vi "Analog_Output_16Channels_W20I5.vi"(1 "Values":fxp<+/-,20,5>[](array[numeric])=[0.0, 0.0, 0.0, 0.0, 0.0, 0.0, 0.0, 0.0, 0.0, 0.0, 0.0, 0.0, 0.0, 0.0, 0.0, 0.0], 2 "IO":T1={"AO 0"="Mod4/AO0", "AO 1"="Mod4/AO0", "AO 2"="Mod4/AO0", "AO 3"="Mod4/AO0", "AO 4"="Mod4/AO0", "AO 5"="Mod4/AO0", "AO 6"="Mod4/AO0", "AO 7"="Mod4/AO0", "AO 8"="Mod4/AO0", "AO 9"="Mod4/AO0", "AO 10"="Mod4/AO0", "AO 11"="Mod4/AO0", "AO 12"="Mod4/AO0", "AO 13"="Mod4/AO0", "AO 14"="Mod4/AO0", "AO 15"="Mod4/AO0"}) -> ()   [LabVIEW 2015]
uses:
  <vilib>/rvi/eio/common/nirviEmuTemplateMethod_errors.vi
  <vilib>/eio/EIONode/EIONode.xnode
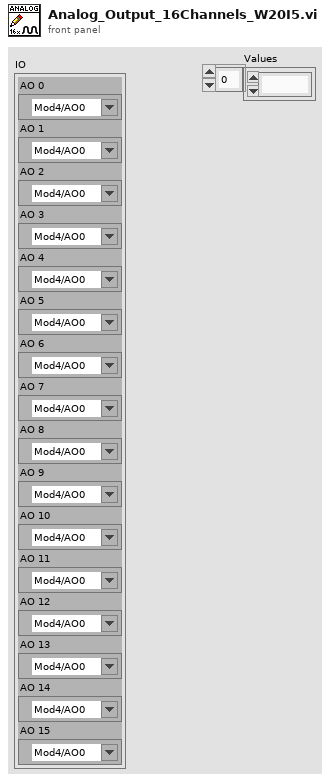
[diagram p1: front panel]
types:
  T1 = cluster{"AO 0":refnum<k21>, "AO 1":refnum<k21>, "AO 2":refnum<k21>, "AO 3":refnum<k21>, "AO 4":refnum<k21>, "AO 5":refnum<k21>, "AO 6":refnum<k21>, "AO 7":refnum<k21>, "AO 8":refnum<k21>, "AO 9":refnum<k21>, "AO 10":refnum<k21>, "AO 11":refnum<k21>, "AO 12":refnum<k21>, "AO 13":refnum<k21>, "AO 14":refnum<k21>, "AO 15":refnum<k21>}
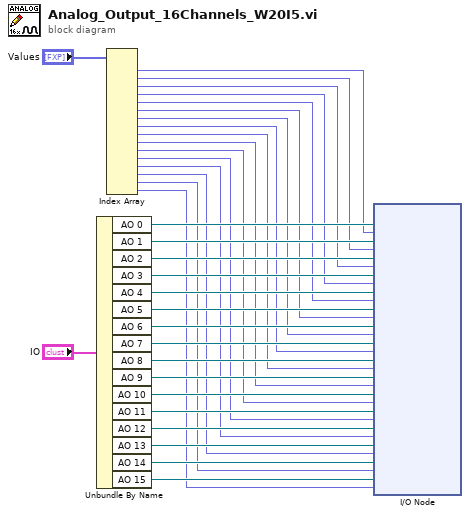
[diagram p0: block diagram]
diagram:
  n1 = Unbundle By Name("IO") -> ("AO 0"=w33:refnum<k21>, "AO 1"=w32:refnum<k21>, "AO 2"=w31:refnum<k21>, "AO 3"=w30:refnum<k21>, "AO 4"=w29:refnum<k21>, "AO 5"=w28:refnum<k21>, "AO 6"=w27:refnum<k21>, "AO 7"=w26:refnum<k21>, "AO 8"=w25:refnum<k21>, "AO 9"=w24:refnum<k21>, "AO 10"=w23:refnum<k21>, "AO 11"=w22:refnum<k21>, "AO 12"=w21:refnum<k21>, "AO 13"=w20:refnum<k21>, "AO 14"=w19:refnum<k21>, "AO 15"=w18:refnum<k21>)
  n2 = Index Array(array="Values") -> (element #1=w16:fxp<+/-,20,5>, element #2=w15:fxp<+/-,20,5>, element #3=w14:fxp<+/-,20,5>, element #4=w13:fxp<+/-,20,5>, element #5=w12:fxp<+/-,20,5>, element #6=w11:fxp<+/-,20,5>, element #7=w10:fxp<+/-,20,5>, element #8=w9:fxp<+/-,20,5>, element #9=w8:fxp<+/-,20,5>, element #10=w7:fxp<+/-,20,5>, element #11=w6:fxp<+/-,20,5>, element #12=w5:fxp<+/-,20,5>, element #13=w4:fxp<+/-,20,5>, element #14=w3:fxp<+/-,20,5>, element #15=w2:fxp<+/-,20,5>, element #16=w1:fxp<+/-,20,5>)  [unwired: 16 in]
  n3 = xnode "I/O Node"("I/O Item"=w16, "FPGA I/O In"=w33, "I/O Item"=w15, "FPGA I/O In"=w32, "I/O Item"=w14, "FPGA I/O In"=w31, "I/O Item"=w13, "FPGA I/O In"=w30, "I/O Item"=w12, "FPGA I/O In"=w29, "I/O Item"=w11, "FPGA I/O In"=w28, "I/O Item"=w10, "FPGA I/O In"=w27, "I/O Item"=w9, "FPGA I/O In"=w26, "I/O Item"=w8, "FPGA I/O In"=w25, "I/O Item"=w7, "FPGA I/O In"=w24, "I/O Item"=w6, "FPGA I/O In"=w23, "I/O Item"=w5, "FPGA I/O In"=w22, "I/O Item"=w4, "FPGA I/O In"=w21, "I/O Item"=w3, "FPGA I/O In"=w20, "I/O Item"=w2, "FPGA I/O In"=w19, "I/O Item"=w1, "FPGA I/O In"=w18) -> ()  [unwired: 16 out]
